vi "Close.vi"(8 "error in (no error)":errorcluster, 11 "FTP in":refnum<class "FTP.lvclass">) -> (0 "error out":errorcluster)   [LabVIEW 2014, in "FTP.lvlib" / "FTP.lvclass"]
doc: "This vi will disconnect from the FTP Server if a connection is detected, and destroy any data that is being held in memory from the FTP Toolkit."
uses:
  FTP.lvclass
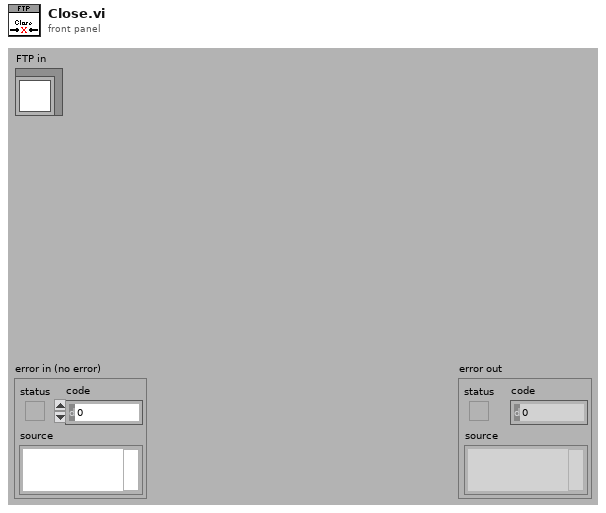
[diagram p1: front panel]
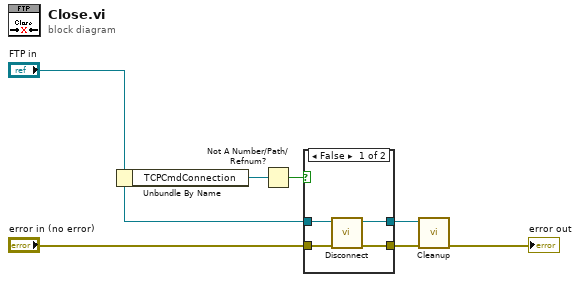
[diagram p0: block diagram]
diagram:
  n1 = Unbundle By Name("FTP in") -> ("TCPCmdConnection"=w2:refnum<k5>)
  n2 = Not A Number/Path/Refnum?(number/path/refnum=w2) -> (NaN/Path/Refnum?=w1:bool)
  n3 = case shown="False" w1 {
    tunnel: "error in (no error)" -> [w11 w12]
    tunnel: [w10 w12] -> w5
    tunnel: [w9 w13] -> w4
    tunnel: "FTP in" -> [w8 w13]
    frame False {
      n4 = call "Disconnect.vi"("error in (no error)"=w11, "FTP in"=w8) -> ("error out"=w10:errorcluster, "FTP out"=w9:refnum<class "FTP.lvclass">)  [unwired: 8 in]
    }
    frame True {
    }
  }
  n5 = call "Cleanup.vi"("error in (no error)"=w5, "FTP in"=w4) -> ("error out"=→"error out":errorcluster)  [unwired: 8 in, 1 out]
